vi "Pack for gRPC.vi"(8 "error in":errorcluster, 9 "configuration / results":enum16{"Configuration", "Results"}(ring), 10 "data value":variant, 11 "measurement customizations in":refnum<class "Measurement Plugin.lvclass">) -> (0 "error out":errorcluster, 2 "any":T1, 3 "measurement customizations out":refnum<class "Measurement Plugin.lvclass">)   [LabVIEW 2021, in "Short-Circuit.lvlib" / "Measurement Plugin.lvclass"]
uses:
  Measurement Plugin.lvclass
  <vilib>/gRPC/LabVIEW gRPC Library/Shared/Any.ctl
  C:/Program Files/National Instruments/LabVIEW 2021/vi.lib/Plug-In SDKs/Measurements/Measurement Plugin Service/Measurement Plugin Service.lvclass
  Measurement Configuration.ctl
  Measurement Results.ctl
  2eca732d-dbaa-43bf-a7dd-ede2da65bc1b.vi
  a6012965-5700-4384-8228-972e71b6560c.vi
  <vilib>/gRPC/LabVIEW gRPC Library/Server API/Translate Protobuf Error.vi
  <vilib>/AdvancedString/1D String Array to Delimited String.vi
  <vilib>/gRPC/LabVIEW gRPC Library/Server API/Server/Get Server DLL Path.vi
  Measurement Plugin.lvclass/Measurement Plugin.ctl
  Short-Circuit.lvlib
  <vilib>/Plug-In SDKs/Measurements/Measurement Plugin Service/Measurement Plugin Service.lvclass
  <vilib>/gRPC/LabVIEW gRPC Library/grpc-lvsupport-release.lvlib
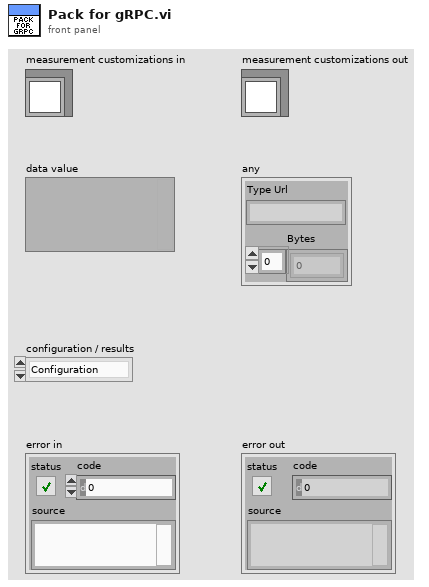
[diagram p1: front panel]
types:
  T1 = typedef "grpc-lvsupport-release.lvlib/Any.ctl" = cluster{"Type Url":string, "Bytes":u8[]}
  T2 = typedef "grpc-lvsupport-release.lvlib/grpcId.ctl" = u64
  T3 = typedef "Short-Circuit.lvlib/Measurement Configuration.ctl" = cluster{"DUT setup time":dbl, "Source delay":dbl, "Aperture time":dbl, "Source resource name":string, "Source sense":i32, "Source current limit":dbl, "Source maximum power":dbl, "Source Voltage (Vo)":dbl, "Load resource name":string, "Load sense":i32, "Load voltage limit range":dbl, "Load Voltage Limit":dbl, "Load Current Level (Io)":dbl, "Switch resource name":string, "Switch - Load Relay Name":string, "Switch - DMM Relay Name":string, "Relay Topology":string, "DMM resource name":string, "DMM Current Range(A)":dbl, "SC - Trigger Delay (sec)":dbl, "SC - Hold Delay (sec)":dbl, "Resolution in Digits":dbl}
  T4 = typedef "Short-Circuit.lvlib/Measurement Results.ctl" = cluster{"Status":string, "Source voltages":dbl[], "Load voltages":dbl[], "Source Current":dbl[], "Load Current":dbl[]}
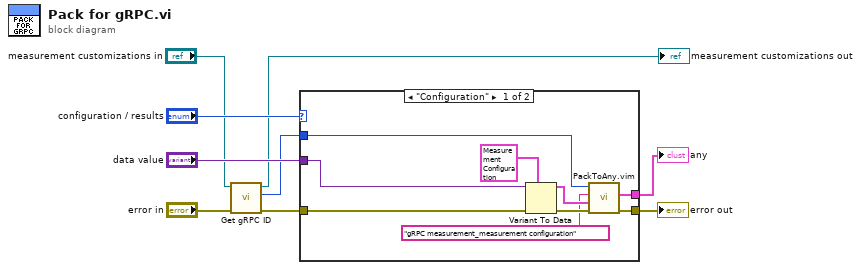
[diagram p0: block diagram]
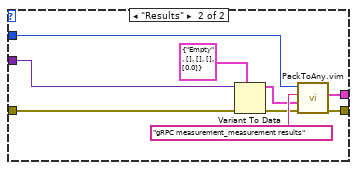
[diagram p2: hidden frame]
diagram:
  n1 = call <vilib>:"Get gRPC ID.vi"("error in"="error in", "measurement plugin service in"="measurement customizations in") -> ("error out"=w4:errorcluster, "gRPC ID"=w1:T2, "measurement plugin service out"=→"measurement customizations out":refnum<class "Measurement Plugin.lvclass">)  [unwired: 7 in]
  n2 = case shown="\"Configuration\"" "configuration / results" {
    tunnel: w4 -> [w18 w27]
    tunnel: "data value" -> [w17 w26]
    tunnel: w1 -> [w14 w22]
    tunnel: [w16 w24] -> w8
    tunnel: [w15 w23] -> w7
    frame "Configuration" {
      n3 = Variant To Data(error in=w18, type=T3 {"DUT setup time"=1.2, "Source delay"=1.2, "Aperture time"=32.0, "Source resource name"="Lorem ipsum dolor sit", "Source sense"=64, "Source current limit"=64.0, "Source maximum power"=-32.0, "Source Voltage (Vo)"=-32.0, "Load resource name"="", "Load sense"=-64, "Load voltage limit range"=1.0, "Load Voltage Limit"=1.0, "Load Current Level (Io)"=1.0, "Switch resource name"="", "Switch - Load Relay Name"="", "Switch - DMM Relay Name"="", "Relay Topology"="Configured Topology", "DMM resource name"="", "DMM Current Range(A)"=0.1, "SC - Trigger Delay (sec)"=0.1, "SC - Hold Delay (sec)"=0.1, "Resolution in Digits"=5.5} ("measurement configuration"), Variant=w17) -> (data=w13:T3, error out=w12:errorcluster)
      n4 = call "PackToAny.vim"("error in"=w12, "Data To Pack"=w13, "Message Type"="gRPC measurement_measurement configuration", "gRPCid in"=w14) -> ("error out"=w16:errorcluster, "Any"=w15:T1)  [unwired: 5 in, 1 out]
    }
    frame "Results" {
      n5 = Variant To Data(error in=w27, type=T4 {"Status"="Empty", "Source voltages"=[], "Load voltages"=[], "Source Current"=[], "Load Current"=[0.0]} ("Measurement Results"), Variant=w26) -> (data=w20:T4, error out=w19:errorcluster)
      n6 = call "PackToAny.vim"("error in"=w19, "Data To Pack"=w20, "Message Type"="gRPC measurement_measurement results", "gRPCid in"=w22) -> ("error out"=w24:errorcluster, "Any"=w23:T1)  [unwired: 5 in, 1 out]
    }
  }
  "error out" <- w8
  "any" <- w7
